vi "PH_AWG-510.read Trigger Settings from String Data File.vi"(1 "Data File String":string) -> (0 "Trigger Settings":T2)   [LabVIEW 2014, in "PH_AWG-510.lvlib"]
uses:
  PH_AWG-510.lvlib
  PH_AWG-510.Trigger Settings.ctl
panel:
  in  "Current Settings.Trigger.Mode":T1(ring)
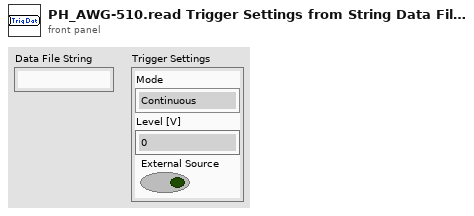
[diagram p1: front panel]
types:
  T1 = enum16{"Continuous", "Triggered", "Gated", "Enhanced"}
  T2 = typedef "PH_AWG-510.lvlib/PH_AWG-510.Trigger Settings.ctl" = cluster{"Mode":enum16{"Continuous", "Triggered", "Gated", "Enhanced"}, "Level (V)":dbl, "External Source":bool}
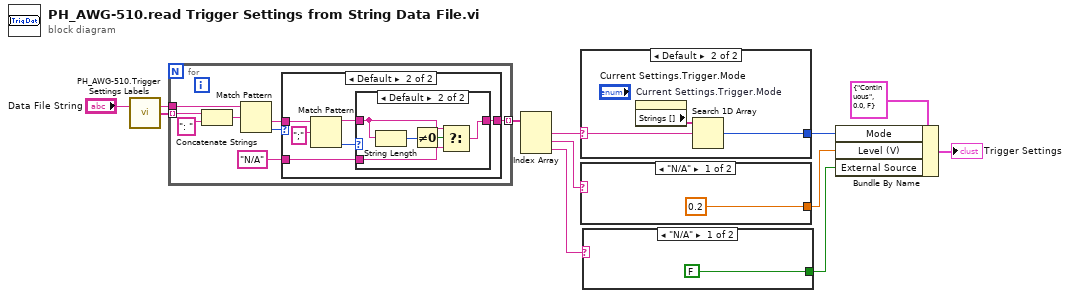
[diagram p0: block diagram]
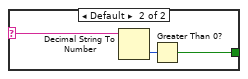
[diagram p4: hidden frame]
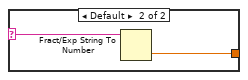
[diagram p5: hidden frame]
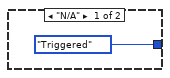
[diagram p6: hidden frame]
diagram:
  n1 = call "PH_AWG-510.Trigger Settings Labels.vi"() -> ("Trigger Settings Labels"=w3:string[])
  n2 = for {
    tunnel: "Data File String" -> [w19]
    tunnel: w3 -> [w17] mode=indexing
    tunnel: [w13] -> w1 mode=indexing
    n3 = Concatenate Strings(w17, ": " ("string")) -> (w18:string)
    n4 = Match Pattern(string=w19, regular expression=w18) -> (after substring=w14:string, offset past match=w15:i32)  [unwired: 1 in, 2 out]
    n5 = case shown="Default" w15 {
      tunnel: w14 -> [_ w26]
      tunnel: [w20 w23] -> w13
      tunnel: "N/A" -> [w20 w21]
      frame -1 {
      }
      frame Default {
        n6 = Match Pattern(string=w26, regular expression=";") -> (before substring=w22:string, offset past match=w24:i32)  [unwired: 1 in, 2 out]
        n7 = case shown="Default" w24 {
          tunnel: [w27 w28] -> w23
          tunnel: w22 -> [_ w30]
          tunnel: w21 -> [w27 w29]
          frame -1 {
          }
          frame Default {
            n8 = String Length(string=w30) -> (length=w32:i32)
            n9 = Not Equal To 0?(x=w32) -> (x != 0?=w31:bool)
            n10 = Select(t=w30, s=w31, f=w29) -> (s? t:f=w28:string)
          }
        }
      }
    }
  }
  n11 = Index Array(array=w1) -> (element #1=w7:string, element #2=w5:string, element #3=w4:string)  [unwired: 3 in]
  n12 = case shown="Default" w7 {
    selector: w7 -> [_ w34]
    tunnel: [T1."Triggered" ("Mode") w35] -> w6
    frame "N/A" {
    }
    frame Default {
      n13 = property on="Current Settings.Trigger.Mode" class="Enum (strict)"() -> ("Strings []"=w36:string[])  [unwired: 2 in, 2 out]
      n14 = Search 1D Array(1D array=w36, element=w34) -> (index of element=w35:i32)  [unwired: 1 in]
    }
  }
  n15 = case shown="\"N/A\"" w5 {
    selector: w5 -> [_ w38]
    tunnel: [0.2 w39] -> w8
    frame "N/A" {
    }
    frame Default {
      n16 = Fract/Exp String To Number(string=w38) -> (number=w39:dbl)  [unwired: 3 in, 1 out]
    }
  }
  n17 = case shown="\"N/A\"" w4 {
    selector: w4 -> [_ w41]
    tunnel: [FALSE w42] -> w9
    frame "N/A" {
    }
    frame Default {
      n18 = Decimal String To Number(string=w41) -> (number=w43:i32)  [unwired: 2 in, 1 out]
      n19 = Greater Than 0?(x=w43) -> (x > 0?=w42:bool)
    }
  }
  n20 = Bundle By Name(cluster=T2 {"Mode"=enum."Continuous", "Level (V)"=0.0, "External Source"=FALSE} ("Trigger Settings"), "Mode"=w6, "Level (V)"=w8, "External Source"=w9) -> (→"Trigger Settings":T2)
